vi "Add Routing Channel.vi"(6 "Description":string, 8 "error in (no error)":errorcluster, 9 "States and Connections":T1, 10 "Channel Name":string, 11 "Routes Ref in":T4 format="%.0x") -> (0 "error out":errorcluster, 2 "Channel Ref":T4 format="%.0x", 3 "Routes Ref out":T4 format="%.0x")   [LabVIEW 2017, in "Switch Scripting.lvlib"]
uses:
  Switch Scripting.lvlib
  <vilib>/NI Veristand/Custom Device API/Custom Device Item Ref.ctl
  Shared/Channel States.ctl
  Shared/Routing State.ctl
  Shared/Connection.ctl
  <vilib>/NI Veristand/Custom Device API/Custom Device Channel.ctl
  <vilib>/NI Veristand/Custom Device API/Custom Device Channel Type.ctl
  <vilib>/NI VeriStand/Custom Device API/Custom Device API.lvlib
  Shared/Routing and Faulting Shared.lvlib
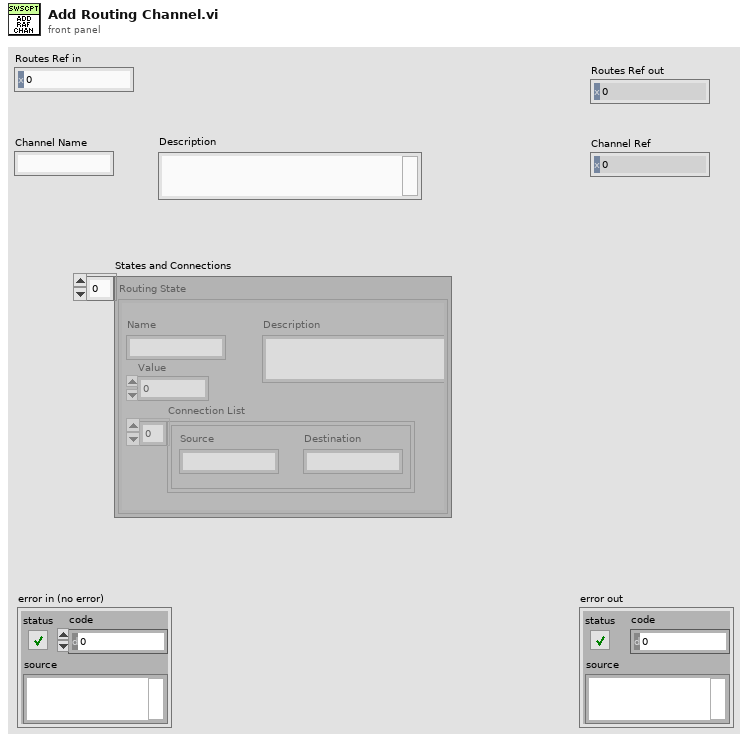
[diagram p1: front panel]
types:
  T1 = typedef "Routing and Faulting Shared.lvlib/Channel States.ctl" = T2[]
  T2 = typedef "Routing and Faulting Shared.lvlib/Routing State.ctl" = cluster{"Name":string, "Description":string, "Value":i32, "Connection List":T3[]}
  T3 = typedef "Routing and Faulting Shared.lvlib/Connection.ctl" = cluster{"Source":string, "Destination":string}
  T4 = typedef "Custom Device API.lvlib/Custom Device Item Ref.ctl" = u64
  T5 = typedef "Custom Device API.lvlib/Custom Device Channel.ctl" = cluster{"Type":T6, "Units":string, "Default Value":dbl, "Faultable":bool, "Scalable":bool}
  T6 = typedef "Custom Device API.lvlib/Custom Device Channel Type.ctl" = enum16{"Input", "Output"}
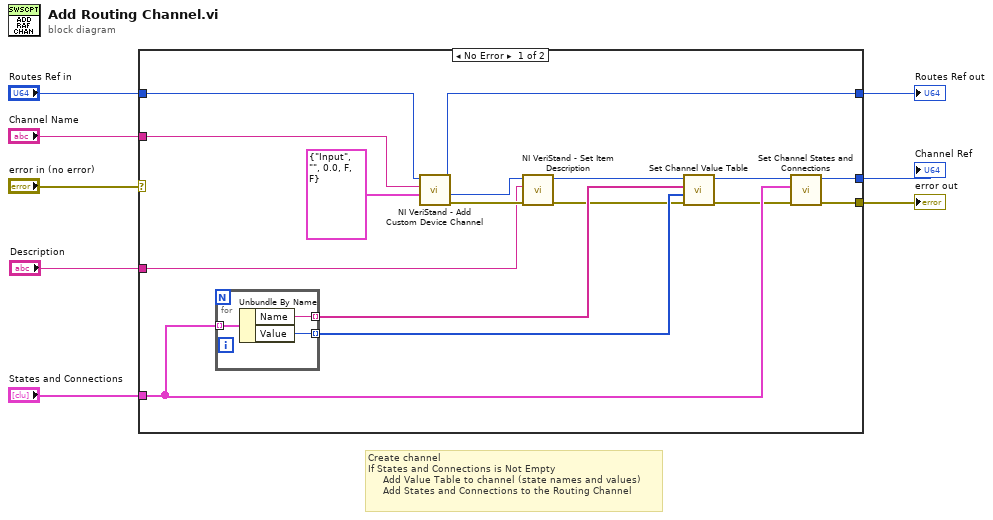
[diagram p0: block diagram]
diagram:
  # "Create channel\nIf States and Connections is Not Empty\n     Add Value Table to channel (state names and values)\n     Add States and Connections to the Routing Channel"
  n1 = case shown="No Error" "error in (no error)" {
    selector: "error in (no error)" -> [_ w29]
    tunnel: [w23 w29] -> w8
    tunnel: [w19 w28] -> w7
    tunnel: "Routes Ref in" -> [w20 w28]
    tunnel: "Channel Name" -> [w24 _]
    tunnel: [w21 _] -> w3
    tunnel: "States and Connections" -> [w22 _]
    tunnel: "Description" -> [w11 _]
    frame No Error {
      n2 = for {
        tunnel: w22 -> [w27] mode=indexing
        tunnel: [w26] -> w16 mode=indexing
        tunnel: [w25] -> w15 mode=indexing
        n3 = Unbundle By Name(w27) -> ("Name"=w26:string, "Value"=w25:i32)
      }
      n4 = call <vilib>:"NI VeriStand - Add Custom Device Channel.vi"("Channel"=T5 {"Type"=enum."Input", "Units"="", "Default Value"=0.0, "Faultable"=FALSE, "Scalable"=FALSE}, "Channel Name"=w24, "Parent Ref in"=w20) -> ("error out"=w13:errorcluster, "Channel Ref"=w10:T4, "Parent Ref out"=w19:T4)  [unwired: 5 in, 1 out]
      n5 = call <vilib>:"NI VeriStand - Set Item Description.vi"("error in (no error)"=w13, "Description"=w11, "Item Ref in"=w10) -> ("error out"=w12:errorcluster, "Item Ref out"=w9:T4)  [unwired: 6 in, 1 out]
      n6 = call "Set Channel Value Table.vi"("error in (no error)"=w12, "Values"=w15, "States"=w16, "Channel Ref in"=w9) -> ("error out"=w18:errorcluster, "Channel Ref out"=w14:T4)  [unwired: 6 in]
      n7 = call "Set Channel States and Connections.vi"("error in (no error)"=w18, "Routing Channel States"=w22, "Channel Ref in"=w14) -> ("error out"=w23:errorcluster, "Channel Ref out"=w21:T4)  [unwired: 7 in]
    }
    frame Error {
    }
  }
  "error out" <- w8
  "Routes Ref out" <- w7
  "Channel Ref" <- w3
